vi "Test Process Multiple Parallell Processes.vi"(8 "error in (no error)":errorcluster, 11 "Rig Test In":refnum<class "Process Test.lvclass">) -> (0 "error out":errorcluster, 3 "Rig Test Out":refnum<class "Process Test.lvclass">)   [LabVIEW 2020, in "Process Test.lvclass"]
uses:
  Process Test.lvclass
  C:/Program Files (x86)/National Instruments/LabVIEW 2020/vi.lib/Asteme/LUnit/Test Case.lvclass
  Mock Error Handler/Mock Error Handler.lvclass
  C:/Users/anton/Documents/GitHub/Triarc-Framework/source/Framework/Error Handler Interface/Error Handler Interface.lvclass
  Framework/Process/Process.lvclass/Process.ctl
  <vilib>/Asteme/LUnit/Test Case.lvclass/Test Case.ctl
  <vilib>/Asteme/LUnit/LUnit Assertion Result.lvclass/LUnit Assertion Result.ctl
  Framework/Process/Public/Lifecycle/Get Lifecycle State.vi
  Framework/Process/Protected/Messaging/Enqueue Message.vi
  <vilib>/Utility/error.llb/Clear Errors.vi
  Framework/Process/Private/SubVIs/Wait for finish.vi
  Framework/Process/Private/SubVIs/Set Lifecycle State.vi
  <vilib>/Asteme/LUnit/Palette/Pass If.vi
  <vilib>/Asteme/LUnit/Set Assertion Type.vi
  <vilib>/Asteme/LUnit/Palette/Pass.vi
  <vilib>/Asteme/LUnit/Palette/Fail.vi
  <vilib>/Asteme/LUnit/LUnit Write Assertion Type.vi
  <vilib>/Asteme/LUnit/Add test result.vi
  <vilib>/Asteme/LUnit/LUnit Write Passed.vi
  <vilib>/Asteme/LUnit/LUnit Get Test Case.vi
  <vilib>/Asteme/LUnit/Assertion Result/LUnit Get Test Name.vi
  <vilib>/Asteme/LUnit/LUnit Write Message.vi
  <vilib>/Asteme/LUnit/LUnit Write Description.vi
  <vilib>/Asteme/LUnit/Read Test Case Name.vi
  <vilib>/Utility/error.llb/Error Cluster From Error Code.vi
  Framework/Process/Process.lvclass
  <vilib>/Asteme/LUnit/LUnit Assertion Result.lvclass
  <vilib>/Asteme/LUnit/Test Case.lvclass
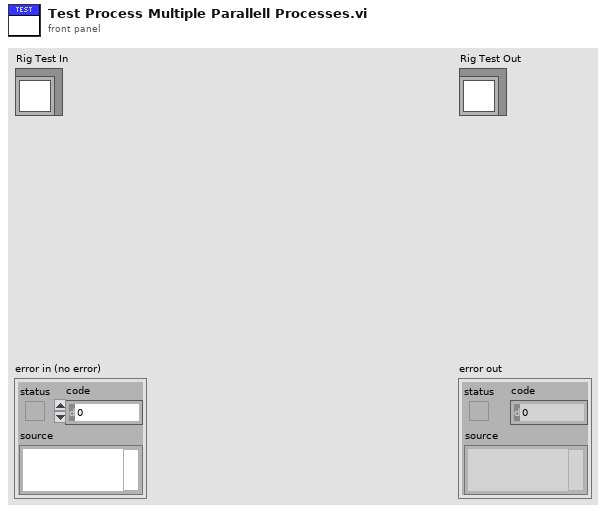
[diagram p1: front panel]
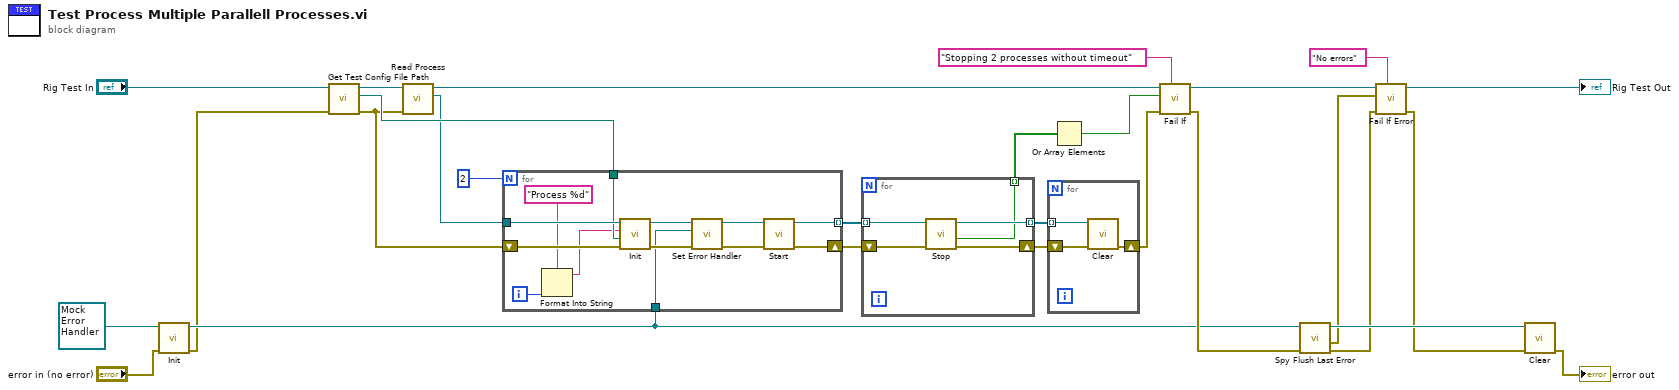
[diagram p0: block diagram]
diagram:
  n1 = call-dynamic "Init.vi"("error in (no error)"="error in (no error)", "Mock Error Handler In"=refnum<class "Mock Error Handler.lvclass"> refnum ("Mock Error Handler.lvclass")) -> ("error out"=w2:errorcluster, "Mock Error Handler Out"=w9:refnum<class "Mock Error Handler.lvclass">)  [unwired: 8 in]
  n2 = call-dynamic "Get Test Config File Path.vi"("error in (no error)"=w2, "Base Class Test in"="Rig Test In") -> ("error out"=w1:errorcluster, "Test config path"=w4:path, "Base Class Test out"=w6:refnum<class "Process Test.lvclass">)  [unwired: 7 in]
  n3 = call "Read Process.vi"("error in (no error)"=w1, "Process Test in"=w6) -> ("Process.lvclass"=w3:refnum<class "Process.lvclass">, "Process Test out"=w7:refnum<class "Process Test.lvclass">)  [unwired: 7 in, 1 out]
  n4 = for {
    N: 2 -> [_]
    tunnel: [w41] -> w26 mode=indexing
    tunnel: w3 -> [w38]
    shift-right: [w40] -> w25
    shift-left: w1 -> [w39]
    tunnel: w9 -> [w33]
    tunnel: w4 -> [w32]
    i -> [w30]
    n5 = Format Into String(format string="Process %d", w30) -> (resulting string=w29:string)  [unwired: 2 in, 1 out]
    n6 = call-dynamic "Init.vi"("error in (no error)"=w39, "Config File Path"=w32, "Name"=w29, "Process In"=w38) -> ("error out"=w35:errorcluster, "Process Out"=w37:refnum<class "Process.lvclass">)  [unwired: 6 in]
    n7 = call "Set Error Handler.vi"("error in (no error)"=w35, "Error Handler"=w33, "Process In"=w37) -> ("error out"=w34:errorcluster, "Process Out"=w36:refnum<class "Process.lvclass">)  [unwired: 7 in]
    n8 = call "Start.vi"("error in (no error)"=w34, "Process In"=w36) -> ("error out"=w40:errorcluster, "Process Out"=w41:refnum<class "Process.lvclass">)  [unwired: 8 in]
  }
  n9 = for {
    tunnel: [w42] -> w22 mode=indexing
    shift-right: [w43] -> w23
    shift-left: w25 -> [w45]
    tunnel: w26 -> [w46] mode=indexing
    tunnel: [w44] -> w24 mode=indexing
    n10 = call "Stop.vi"("error in (no error)"=w45, "Process In"=w46) -> ("error out"=w43:errorcluster, "timed out?"=w42:bool, "Process Out"=w44:refnum<class "Process.lvclass">)  [unwired: 7 in]
  }
  n11 = for {
    tunnel: w24 -> [w49] mode=indexing
    shift-right: [w47] -> w19
    shift-left: w23 -> [w48]
    n12 = call-dynamic "Clear.vi"("error in (no error)"=w48, "Process In"=w49) -> ("error out"=w47:errorcluster)  [unwired: 8 in, 1 out]
  }
  n13 = Or Array Elements(Boolean array=w22) -> (logical OR=w20:bool)
  n14 = call <vilib>:"Fail If.vi"("Description"="Stopping 2 processes without timeout", "error in (no error)"=w19, "Fail?"=w20, "Test Case In"=w7) -> ("error out"=w10:errorcluster, "Test Case Out"=w27:refnum<class "Process Test.lvclass">)  [unwired: 6 in]
  n15 = call "Spy Flush Last Error.vi"("error in (no error)"=w10, "Mock Error Handler In"=w9) -> ("error out"=w15:errorcluster, "Error"=w14:errorcluster, "Mock Error Handler Out"=w18:refnum<class "Mock Error Handler.lvclass">)  [unwired: 7 in]
  n16 = call <vilib>:"Fail If Error.vi"("Description"="No errors", "error in (no error)"=w15, "Assert error"=w14, "Test Case In"=w27) -> ("error out"=w12:errorcluster, "Test Case Out"=→"Rig Test Out":refnum<class "Process Test.lvclass">)  [unwired: 6 in]
  n17 = call-dynamic "Clear.vi"("error in (no error)"=w12, "Mock Process In"=w18) -> ("error out"=→"error out":errorcluster)  [unwired: 8 in, 1 out]
